vi "main-top地址搜索-随机秘钥.vi"() -> ()   [LabVIEW 2020]
uses:
  C:/Program Files (x86)/National Instruments/LabVIEW 2020/examples/Connectivity/Python/support/PythonVersionsEnum.ctl
  86b1dac1-cd05-41a7-bc2f-191b5b3d7e20.vi
  <vilib>/Utility/file.llb/Read Delimited Spreadsheet (string).vi
  <vilib>/Utility/file.llb/Write Delimited Spreadsheet (string).vi
  <vilib>/Comparison/Equal/Equal Functor/Equal Functor.lvclass
panel:
  out "data base":string[](array[string])
  out "添加的路径 4":path
  out "添加的路径 3":path
  out "添加的路径 2":path
  out "eth地址":string
  out "添加的路径":path
  out "find private key":string[][](array[string])
  out "错误输出":errorcluster
  out "私钥":string
  out "已找寻数":i32
  out "添加的数组":string[](array[string])
  out "数值 4":i32
  out "error out 2":cluster{"状态":bool, "代码":i32, "源":string} caption="错误输出"
  in  "error in (no error)":cluster{"状态":bool, "代码":i32, "源":string} caption="错误输入（无错误）"
  out "非压缩地址 2":string
  out "压缩地址 2":string
  in  "停止":bool
  out "文件名":string[](array[string])
  out "路径输出":path
  # "比特币以太坊地址随机比对器"
  # "donation：\neth、bsc、ht、matic Any virtual currency at this address\n0xCEb24266E9A912a89302A46C1E04cD0DFBF751C8"
  # "D:\\NI 资源包\\2-币猎人-事件状态机930\\source\\网址私钥获取\\btc搜寻器1\\python"
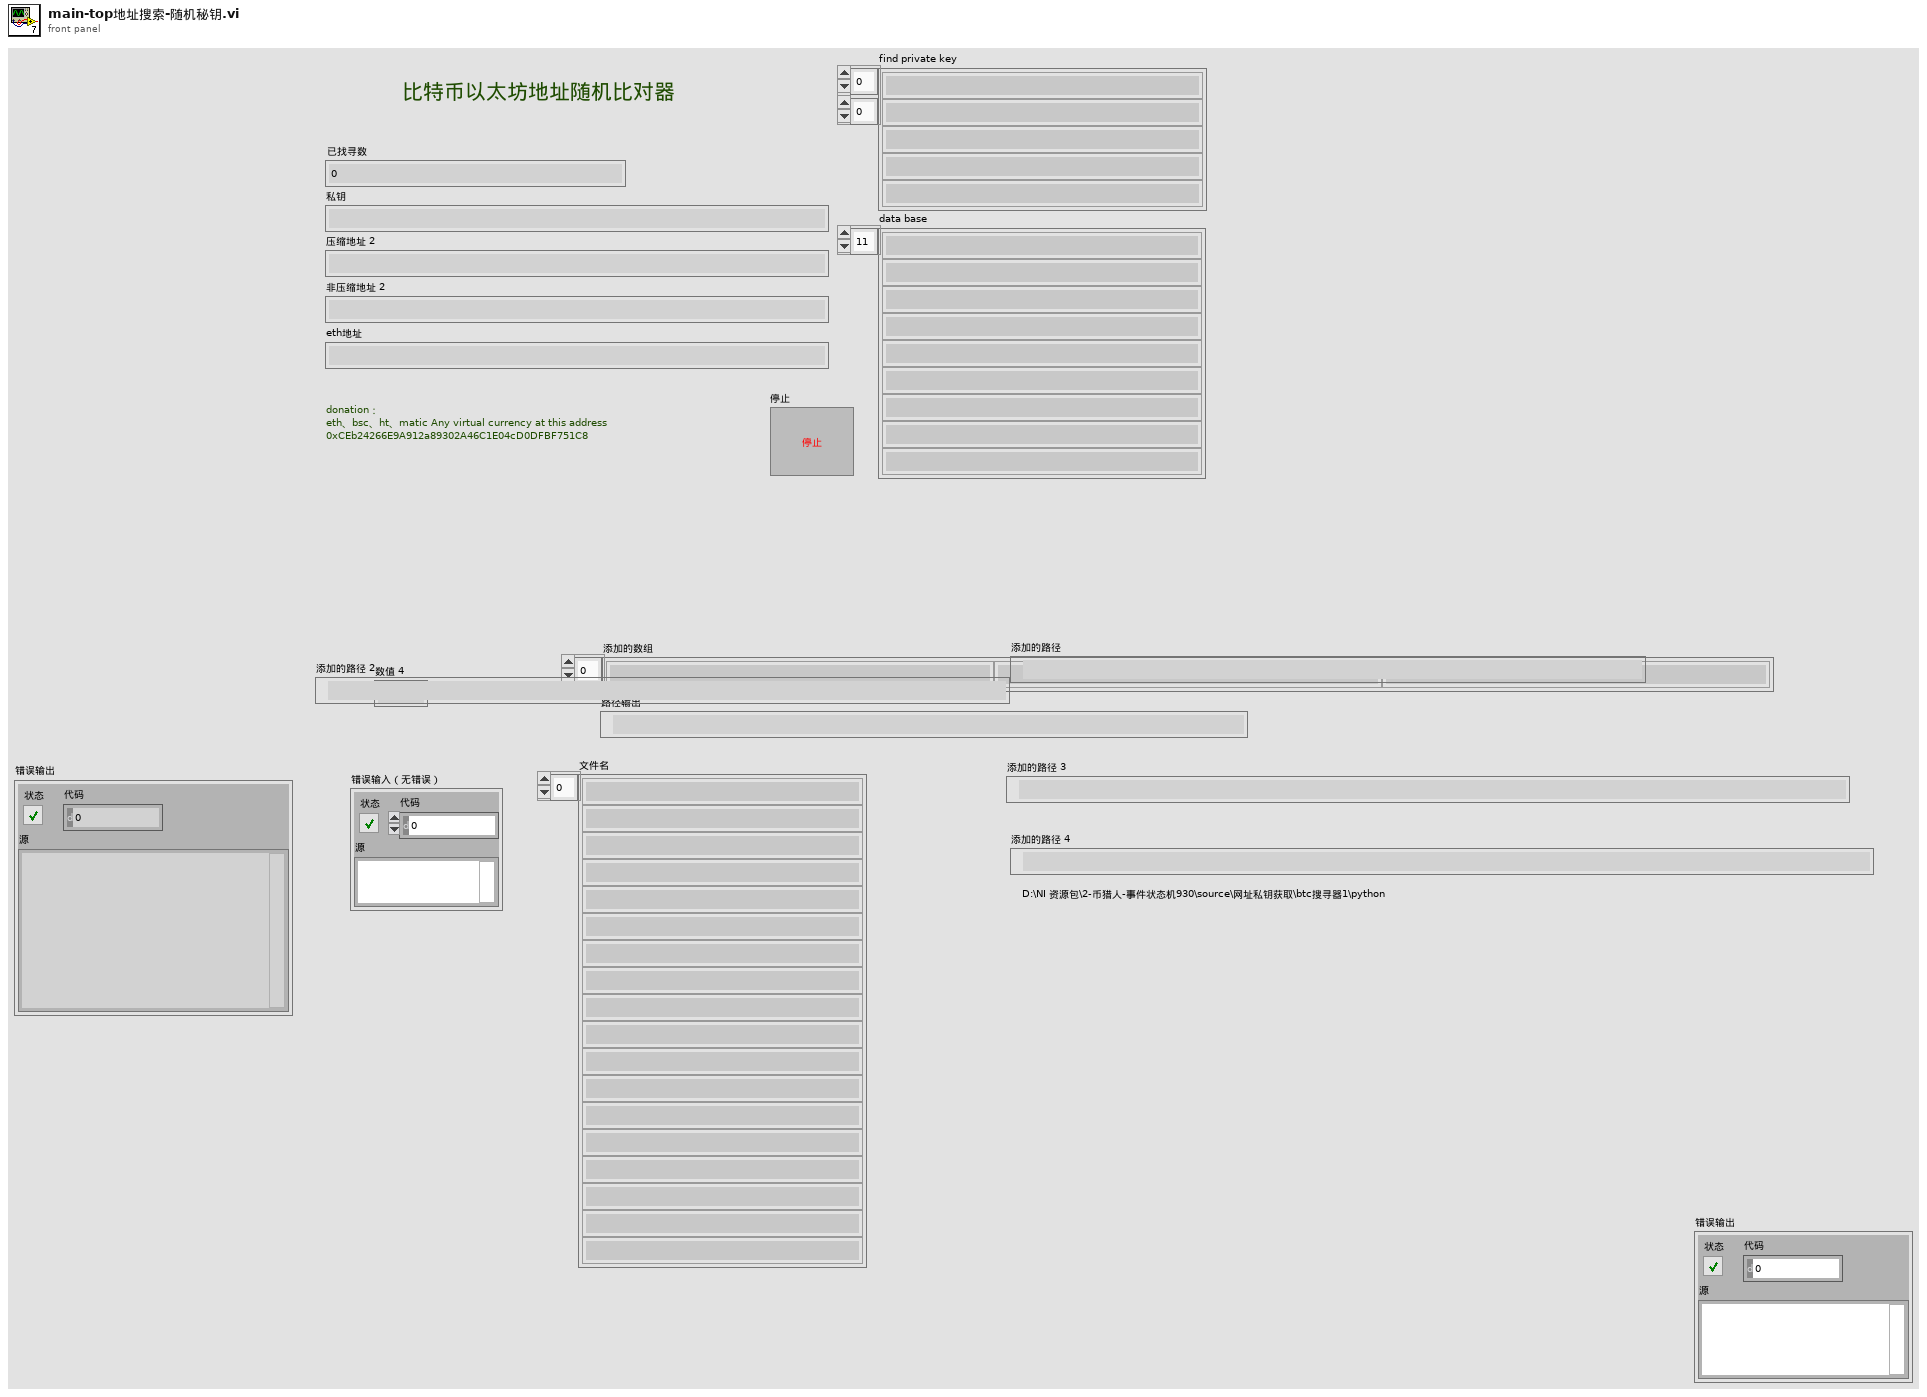
[diagram p1: front panel]
types:
  T1 = typedef "PythonVersionsEnum.ctl" = enum16{"2.7", "3.6"}
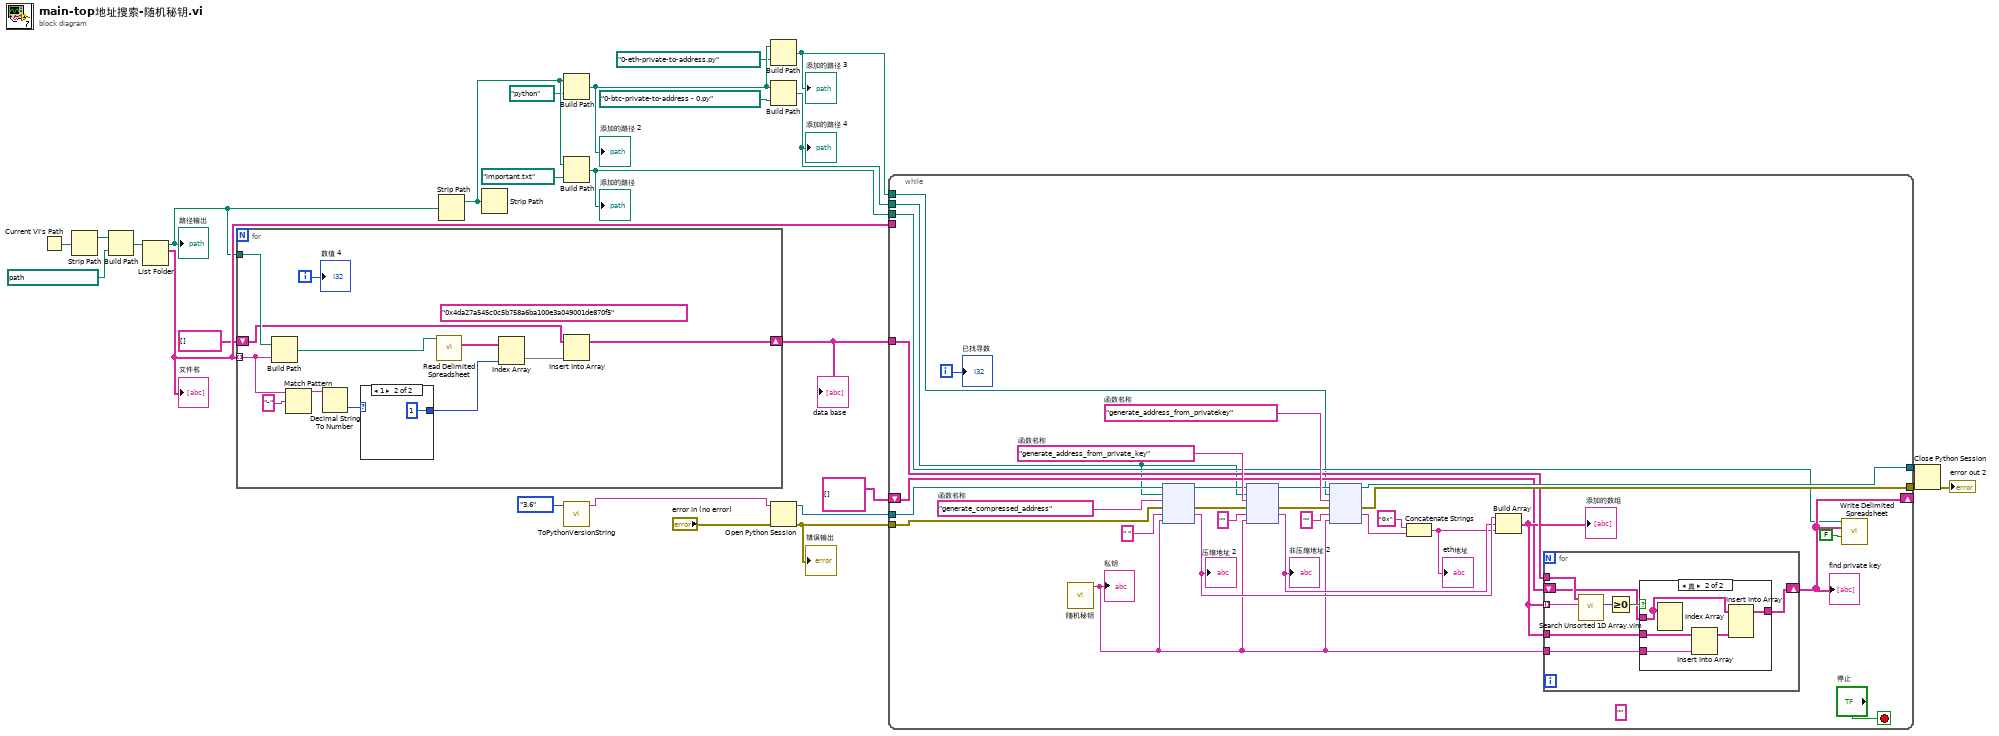
[diagram p0: block diagram]
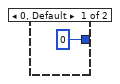
[diagram p2: hidden frame]
diagram:
  n1 = Current VI's Path() -> (path=w9:path)
  n2 = Strip Path(path=w9) -> (stripped path=w8:path)  [unwired: 1 out]
  n3 = Build Path(base path=w8, name or relative path=path "非小号前百位数据" ("名称或相对路径")) -> (appended path=w6:path)
  n4 = List Folder(path=w6) -> (path out=w14:path, filenames=w18:string[])  [unwired: 3 in, 2 out]
  "路径输出" <- w14
  "文件名" <- w18
  n5 = for {
    tunnel: w18 -> [w31] mode=indexing
    tunnel: w14 -> [w30]
    shift-right: [w28] -> w15
    shift-left: string[] [] -> [w27]
    i -> [w32]
    (unwired) "0x4da27a545c0c5b758a6ba100e3a049001de870f5" ("元素 2")
    n6 = Build Path(base path=w30, name or relative path=w31) -> (appended path=w33:path)
    n7 = Match Pattern(string=w31, regular expression="-" ("正则表达式")) -> (before substring=w37:string)  [unwired: 1 in, 3 out]
    n8 = Decimal String To Number(string=w37) -> (number=w36:i32)  [unwired: 2 in, 1 out]
    n9 = case shown="1" w36 {
      tunnel: [0 ("禁用的索引 (列)") 1 ("禁用的索引 (列)")] -> w34
      frame 0, Default {
      }
      frame 1 {
      }
    }
    n10 = call-poly <vilib>:"Read Delimited Spreadsheet.vi"("file path (dialog if empty)"=w33) -> ("all rows"=w35:string[][])  [unwired: 9 in, 5 out]
    n11 = Index Array(array=w35, index (col)=w34) -> (element=w29:string[])  [unwired: 1 in]
    n12 = Insert Into Array(array=w27, new element=w29) -> (w28:string[])  [unwired: 1 in]
    "数值 4" <- w32
  }
  "data base" <- w15
  n13 = Strip Path(path=w14) -> (stripped path=w11:path)  [unwired: 1 out]
  n14 = Strip Path(path=w11) -> ()  [unwired: 2 out]
  n15 = Build Path(base path=w11, name or relative path=path "python" ("名称或相对路径")) -> (appended path=w3:path)
  "添加的路径 2" <- w3
  n16 = Build Path(base path=w11, name or relative path=path "important.txt" ("名称或相对路径")) -> (appended path=w12:path)
  "添加的路径" <- w12
  n17 = call "ToPythonVersionString.vi"("Python版本"=PythonVersionsEnum."3.6") -> ("python版本字符串"=w26:string)  [unwired: 10 in]
  n18 = Build Path(base path=w3, name or relative path=path "0-eth-private-to-address.py" ("名称或相对路径")) -> (appended path=w1:path)
  "添加的路径 3" <- w1
  n19 = Build Path(base path=w3, name or relative path=path "0-btc-private-to-address - 0.py" ("名称或相对路径")) -> (appended path=w4:path)
  "添加的路径 4" <- w4
  n20 = Open Python Session(python version=w26, 3:"error in (no error)") -> (session out=w23:refnum<k35>, error out=w22:errorcluster)  [unwired: 1 in]
  "错误输出" <- w22
  n21 = while {
    tunnel: w18 -> [_]
    tunnel: w23 -> [w55]
    tunnel: w22 -> [w54]
    tunnel: [w53] -> w20
    tunnel: [w52] -> w19
    tunnel: w15 -> [w51]
    shift-right: [w46] -> _
    shift-left: string[][] [] -> [w48]
    tunnel: w12 -> [w45]
    tunnel: w4 -> [w41]
    tunnel: w1 -> [w42]
    i -> [w47]
    stop <- "停止" stop-if-true
    (unwired) "" ("元素")
    w67 = "generate_address_from_privatekey"  # 函数名称
    w68 = "generate_address_from_private_key"  # 函数名称
    w69 = "generate_compressed_address"  # 函数名称
    n22 = call "随机秘钥.vi"() -> ("私钥"=w50:string)  [unwired: 11 in]
    "私钥" <- w50
    n23 = node(w55, w41, w69, w54, " ", w50) -> (w64:refnum<k35>, w63:errorcluster, w57:string)  [unwired: 1 in, 2 out]
    "压缩地址 2" <- w57
    n24 = node(w64, w41, w68, w63, "", w50) -> (w62:refnum<k35>, w61:errorcluster, w56:string)  [unwired: 1 in, 2 out]
    "非压缩地址 2" <- w56
    n25 = node(w62, w42, w67, w61, "", w50) -> (w52:refnum<k35>, w53:errorcluster, w66:string)  [unwired: 1 in, 2 out]
    n26 = Concatenate Strings("0x" ("字符串"), w66) -> (w43:string)
    "eth地址" <- w43
    n27 = Build Array(w57, w56, w43) -> (w49:string[])
    "添加的数组" <- w49
    n28 = for {
      tunnel: w49 -> [w75] mode=indexing
      tunnel: w51 -> [w78]
      tunnel: w50 -> [w74]
      tunnel: w49 -> [w73]
      shift-right: [w71] -> w46
      shift-left: w48 -> [w72]
      n29 = call "Search Unsorted 1D Array.vim"("element"=w75, "unsorted 1D array"=w78) -> ("index of element"=w77:i32)  [unwired: 9 in]
      n30 = Greater Or Equal To 0?(x=w77) -> (x >= 0?=w76:bool)
      n31 = case shown="真" w76 {
        tunnel: w73 -> [_ w84]
        tunnel: w74 -> [_ w83]
        tunnel: w72 -> [w79 w82]
        tunnel: [w79 w81] -> w71
        frame False {
        }
        frame True {
          n32 = Index Array(array=w82) -> ()  [unwired: 2 in, 1 out]
          n33 = Insert Into Array(array=w84, new element=w83) -> (w80:string[])  [unwired: 1 in]
          n34 = Insert Into Array(array=w82, new element=w80) -> (w81:string[][])  [unwired: 2 in]
        }
      }
    }
    "find private key" <- w46
    n35 = call-poly <vilib>:"Write Delimited Spreadsheet.vi"("file path (dialog if empty)"=w45, "2D data"=w46, "append to file? (new file:F)"=FALSE) -> ()  [unwired: 11 in, 2 out]
    "已找寻数" <- w47
  }
  n36 = Close Python Session(session in=w19, error in=w20) -> (11:→"error out 2":errorcluster)
